vi "EndTrial.vi"(8 "error in (no error)":errorcluster, 11 "TrialBasedExperiment in":refnum<class "MatlabExperiment.lvclass">) -> (0 "error out":errorcluster, 3 "TrialBasedExperiment out":refnum<class "MatlabExperiment.lvclass">)   [LabVIEW 2010, in "MatlabExperiment.lvclass"]
uses:
  MatlabExperiment.lvclass
  TrialBasedExperimentObject/TrialBasedExperiment.lvclass
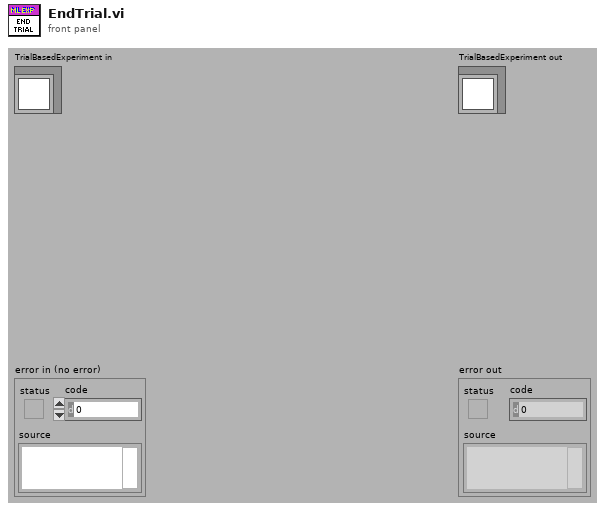
[diagram p1: front panel]
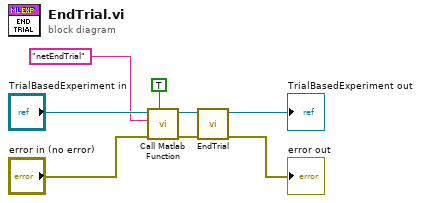
[diagram p0: block diagram]
diagram:
  n1 = call-dynamic "Call Matlab Function.vi"("Timestamp"=TRUE, "error in (no error)"="error in (no error)", "Function name"="netEndTrial", "TrialBasedExperiment in"="TrialBasedExperiment in") -> ("error out"=w4:errorcluster, "TrialBasedExperiment out"=w5:refnum<class "MatlabExperiment.lvclass">)  [unwired: 4 in, 2 out]
  n2 = call-parent "EndTrial.vi"("error in (no error)"=w4, "TrialBasedExperiment in"=w5) -> ("error out"=→"error out":errorcluster, "TrialBasedExperiment out"=→"TrialBasedExperiment out":refnum<class "MatlabExperiment.lvclass">)  [unwired: 8 in]
